vi "carro caña.vi"() -> ()   [LabVIEW 2017]
panel:
  out "Carro_caña":bool
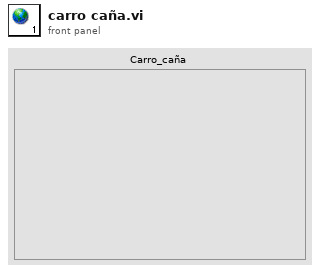
[diagram p1: front panel]
diagram:
